vi "Close.vi"(8 "Error In":errorcluster, 11 "Receiver Ref.":refnum<class "Receiver.lvclass">) -> (0 "Error Out":errorcluster)   [LabVIEW 2020, in "RemoteVariables.lvlib" / "Receiver.lvclass"]
uses:
  Receiver.lvclass
  Receiver.lvclass/Receiver.ctl
  UDP/UDP.lvclass
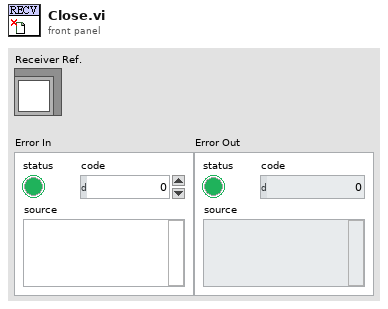
[diagram p1: front panel]
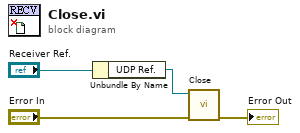
[diagram p0: block diagram]
diagram:
  n1 = Unbundle By Name("Receiver Ref.") -> ("UDP Ref."=w1:refnum<class "UDP.lvclass">)
  n2 = call "Close.vi"("Error In"="Error In", "UDP Ref."=w1) -> ("Error Out"=→"Error Out":errorcluster)  [unwired: 9 in]
